vi "IMA Check and Stop.vi"(0 "IMA Note In":refnum<notifier>, 11 "Error In":errorcluster) -> (4 "IMA Note Out":refnum<notifier>, 15 "Error Out":errorcluster)   [LabVIEW 2020]
uses:
  IMA Type Defs/IMA Actions.ctl
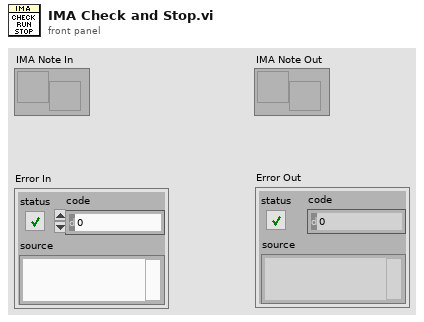
[diagram p1: front panel]
types:
  T1 = typedef "IMA Actions.ctl" = enum16{"Add Position", "Update Saved", "Remove Position", "Capture All", "Capture Here", "Move to Position", "Update Name", "Capture", "Switch", "Clear All", "Abort", "Exit Loop", "Quit"}
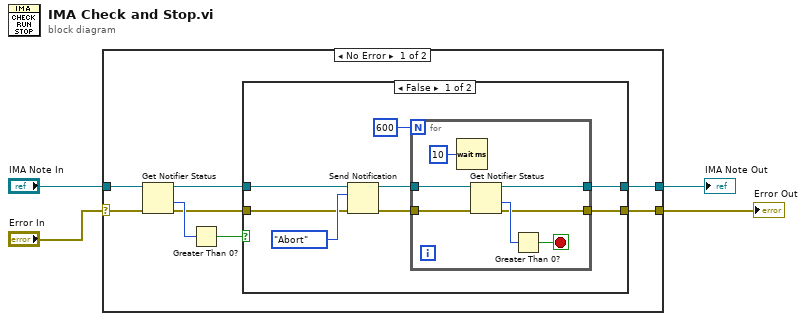
[diagram p0: block diagram]
diagram:
  n1 = case shown="No Error" "Error In" {
    selector: "Error In" -> [w6 w30]
    tunnel: [w8 w31] -> w2
    tunnel: [w7 w30] -> w1
    tunnel: "IMA Note In" -> [w5 w31]
    frame No Error {
      n2 = Get Notifier Status(notifier=w5, error in (no error)=w6) -> (notifier out=w11:refnum<notifier>, # waiting=w12:i32, error out=w9:errorcluster)  [unwired: 2 out]
      n3 = Greater Than 0?(x=w12) -> (x > 0?=w10:bool)
      n4 = case shown="False" w10 {
        tunnel: w11 -> [w17 w29]
        tunnel: w9 -> [w16 w28]
        tunnel: [w15 w29] -> w8
        tunnel: [w13 w28] -> w7
        frame False {
          n5 = Send Notification(notification=IMA_Actions."Abort", notifier=w17, error in (no error)=w16) -> (notifier out=w18:refnum<notifier>, error out=w14:errorcluster)
          n6 = for {
            N: 600 -> [_]
            tunnel: w18 -> [w27]
            tunnel: [w24] -> w15
            tunnel: w14 -> [w22]
            tunnel: [w21] -> w13
            stop <- w25 stop-if-true
            n7 = Wait (ms)(milliseconds to wait=u32 10) -> ()  [unwired: 1 out]
            n8 = Get Notifier Status(notifier=w27, error in (no error)=w22) -> (notifier out=w24:refnum<notifier>, # waiting=w26:i32, error out=w21:errorcluster)  [unwired: 2 out]
            n9 = Greater Than 0?(x=w26) -> (x > 0?=w25:bool)
          }
        }
        frame True {
        }
      }
    }
    frame Error {
    }
  }
  "IMA Note Out" <- w2
  "Error Out" <- w1
